vi "Initialize AI Channels.vi"(8 "error in (no error)":errorcluster, 11 "Instrument.DAQ":refnum<class "Instrument.DAQ.lvclass">) -> (0 "error out":errorcluster, 3 "Instrument.DAQ out":refnum<class "Instrument.DAQ.lvclass">)   [LabVIEW 2019, in "Instrument.Lockin.lvlib" / "Instrument.DAQ.lvclass"]
uses:
  Instrument.DAQ.lvclass
  Instrument.DAQ.lvclass/Instrument.DAQ.ctl
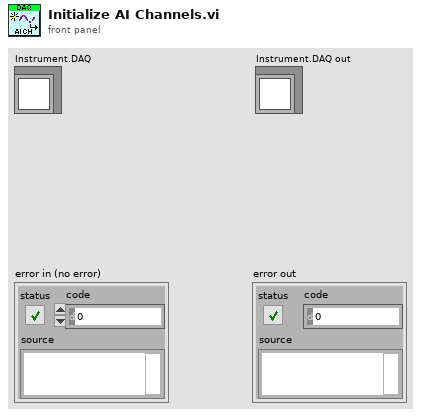
[diagram p1: front panel]
types:
  T1 = typedef "Instrument.Lockin.lvlib/Instrument.DAQ.lvclass/AI.Channel--Cluster--Array.ctl" = T2[]
  T2 = typedef "Instrument.Lockin.lvlib/Instrument.DAQ.lvclass/AI.Channel--Cluster.ctl" = cluster{"Enable?":bool, "Channel":i32, "References":u16[], "reference index":i32}
  T3 = typedef "Instrument.Lockin.lvlib/Instrument.DAQ.lvclass/DAQ.Config.AI--Cluster--Array.ctl" = cluster{"Channels":tag, "Coupling":T4, "Range":T5, "terminal configuration":T6, "Type":T7}[]
  T4 = typedef "Instrument.Lockin.lvlib/Instrument.DAQ.lvclass/DAQ.Config.AI.Coupling--enum.ctl" = u16
  T5 = typedef "Instrument.Lockin.lvlib/Instrument.DAQ.lvclass/DAQ.Config.AI.Range--enum.ctl" = enum16{"±0.316", "±1.00", "±3.16", "±10.0", "±31.6", "±42.4", ""}
  T6 = typedef "Instrument.Lockin.lvlib/Instrument.DAQ.lvclass/DAQ.TerminalConfiguration--ring.ctl" = i32
  T7 = typedef "Instrument.Lockin.lvlib/Instrument.DAQ.lvclass/DAQ.Type--enum.ctl" = enum16{"None", "USB-4431", "PXI-446x"}
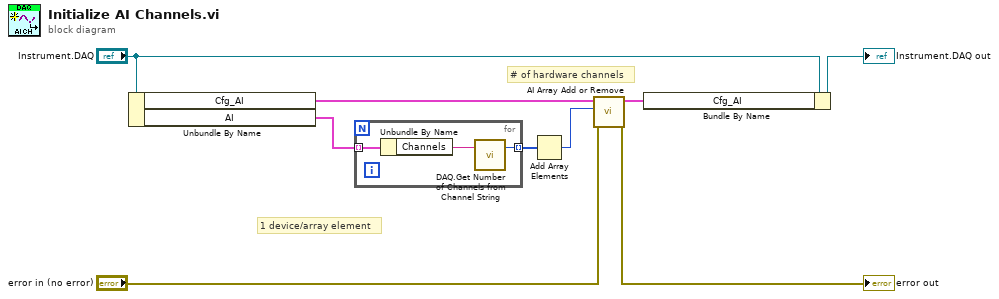
[diagram p0: block diagram]
diagram:
  # "1 device/array element"
  # "# of hardware channels"
  n1 = Unbundle By Name("Instrument.DAQ") -> ("Cfg_AI"=w3:T1, "AI"=w2:T3)
  n2 = for {
    tunnel: w2 -> [w12] mode=indexing
    tunnel: [w11] -> w9 mode=indexing
    n3 = Unbundle By Name(w12) -> ("Channels"=w10:tag)
    n4 = call "DAQ.Get Number of Channels from Channel String.vi"("Channels String"=w10) -> ("# channels"=w11:i32)  [unwired: 2 in]
  }
  n5 = Add Array Elements(numeric array=w9) -> (sum=w1:i32)
  n6 = call "AI Array Add or Remove.vi"("error in (no error)"="error in (no error)", "Size"=w1, "Configuration.Channels.AI"=w3) -> ("error out"=→"error out":errorcluster, "Configuration.Channels.AI"=w6:T1)  [unwired: 7 in]
  n7 = Bundle By Name(cluster="Instrument.DAQ", "Cfg_AI"=w6) -> (→"Instrument.DAQ out":refnum<class "Instrument.DAQ.lvclass">)
